vi "Translate.vi"   [LabVIEW 2015, in "lv-deepl-api.lvlib"]
uses:
  lv-deepl-api.lvlib
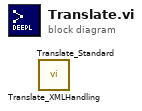
[diagram p0: block diagram]
diagram:
  n1 = call "Translate_XMLHandling.vi"() -> ()  [unwired: 10 in, 2 out]
  n2 = call "Translate_Standard.vi"() -> ()  [unwired: 10 in, 2 out]
